vi "Arrange VIWin - Get Display Workspace Bounds.vi"(11 "error in":errorcluster) -> (4 "display workspace bounds":T1, 15 "error out":errorcluster)   [LabVIEW 2017, in "Arrange VI Window.lvlib"]
uses:
  Arrange VI Window.lvlib
  <resource>/dialog/lvconfig.llb/LV Config Read Numeric (I32).vi
  <vilib>/Utility/miscctls.llb/LVRectTypeDef.ctl
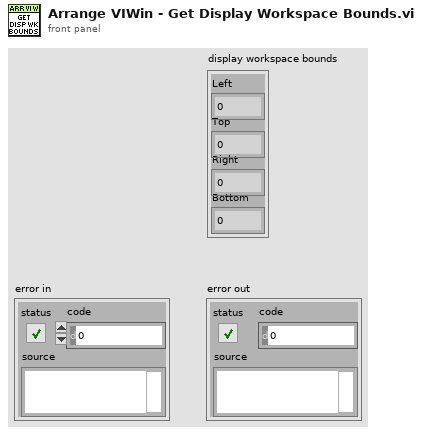
[diagram p1: front panel]
types:
  T1 = typedef "LVRectTypeDef.ctl" = cluster{"Left":i16, "Top":i16, "Right":i16, "Bottom":i16}
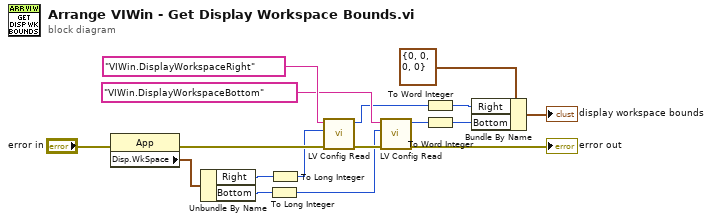
[diagram p0: block diagram]
diagram:
  n1 = property class="App"(error in="error in") -> (error out=w11:errorcluster, "Disp.WkSpace"=w17:T1)  [unwired: 1 in, 1 out]
  n2 = Unbundle By Name(w17) -> ("Right"=w10:i16, "Bottom"=w7:i16)
  n3 = To Long Integer(number=w7) -> (32bit integer=w8:i32)
  n4 = To Long Integer(number=w10) -> (32bit integer=w9:i32)
  n5 = call-poly <resource>:"LV Config Read.vi"("error in"=w11, "default value"=w9, "key"="VIWin.DisplayWorkspaceRight") -> ("error out"=w15:errorcluster, "value"=w12:i32)  [unwired: 2 in, 1 out]
  n6 = call-poly <resource>:"LV Config Read.vi"("error in"=w15, "default value"=w8, "key"="VIWin.DisplayWorkspaceBottom") -> ("error out"=→"error out":errorcluster, "value"=w13:i32)  [unwired: 2 in, 1 out]
  n7 = To Word Integer(number=w12) -> (16bit integer=w5:i16)
  n8 = To Word Integer(number=w13) -> (16bit integer=w4:i16)
  n9 = Bundle By Name(cluster=T1 {"Left"=0, "Top"=0, "Right"=0, "Bottom"=0} ("Display:Primary Workspace"), "Right"=w5, "Bottom"=w4) -> (→"display workspace bounds":T1)
